vi "RegisterSelectionChangeEvent.vi"(0 "reference in":refnum<class "DataGridView.lvclass">, 11 "error in (no error)":errorcluster) -> (4 "reference out":refnum<class "DataGridView.lvclass">, 6 "SelectionChangedEventReg":refnum<event-registration>, 15 "error out":errorcluster)   [LabVIEW 2018, in "DataGridView.lvclass"]
doc: "Registers for the Selection Change event"
uses:
  DataGridView.lvclass
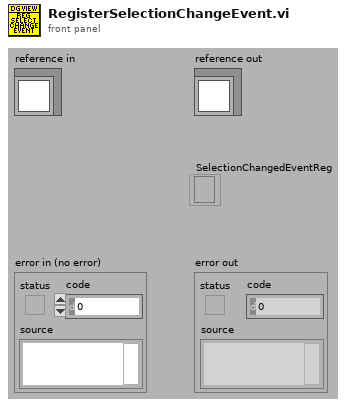
[diagram p1: front panel]
types:
  T1 = typedef "DataGridView.lvclass/ObjectAttributes.ctl" = cluster{"DataGridView":refnum<k24>, "SelectionChangedEvent":refnum<user-event>, "SelectionChanged callback ref":refnum<k27>, "LastSelectedRowIndex":i32, "CellClickEvent":refnum<user-event>, "CellClick callback refnum":refnum<k27>}
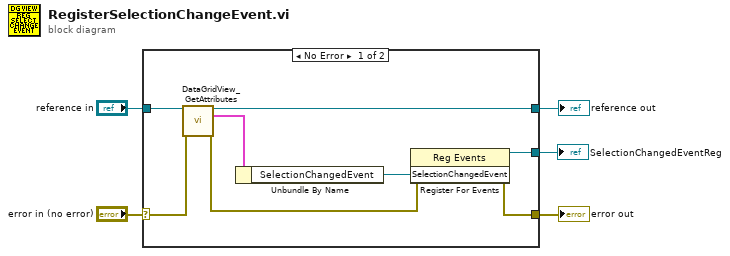
[diagram p0: block diagram]
diagram:
  n1 = case shown="No Error" "error in (no error)" {
    selector: "error in (no error)" -> [w13 w15]
    tunnel: [w8 w15] -> w4
    tunnel: [w10 w14] -> w2
    tunnel: "reference in" -> [w11 w14]
    tunnel: [w9 _] -> w1
    frame No Error {
      n2 = call "DataGridView_GetAttributes.vi"("reference in"=w11, "error in (no error)"=w13) -> ("reference out"=w10:refnum<class "DataGridView.lvclass">, "Data"=w12:T1, "error out"=w6:errorcluster)  [unwired: 10 in, 1 out]
      n3 = Unbundle By Name(w12) -> ("SelectionChangedEvent"=w7:refnum<user-event>)
      n4 = register-events(error in=w6, w7) -> (reference out=w9:refnum<event-registration>, error out=w8:errorcluster)  [unwired: 1 in]
    }
    frame Error {
    }
  }
  "error out" <- w4
  "reference out" <- w2
  "SelectionChangedEventReg" <- w1
